vi "Cleanup.vi"(8 "error in (no error)":errorcluster, 11 "VISA GPS in":refnum<class "VISA GPS.lvclass">) -> (0 "error out":errorcluster)   [LabVIEW 2020, in "nmea.lvlib" / "VISA GPS.lvclass"]
uses:
  VISA GPS.lvclass
  VISA GPS.lvclass/VISA GPS.ctl
  nmea/nmea.lvclass
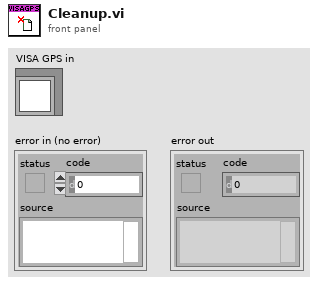
[diagram p1: front panel]
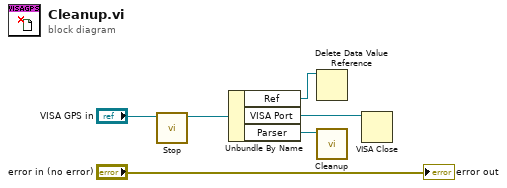
[diagram p0: block diagram]
diagram:
  n1 = call "Stop.vi"("VISA GPS in"="VISA GPS in") -> ("VISA GPS out"=w1:refnum<class "VISA GPS.lvclass">)  [unwired: 9 in, 1 out]
  n2 = Unbundle By Name(w1) -> ("Ref"=w5:refnum<data-value>, "VISA Port"=w4:refnum<visa-resource-name>, "Parser"=w3:refnum<class "nmea.lvclass">)
  n3 = Delete Data Value Reference(data value reference=w5) -> ()  [unwired: 1 in, 2 out]
  n4 = call "Cleanup.vi"("nmea in"=w3) -> ()  [unwired: 10 in, 1 out]
  n5 = VISA Close(VISA resource name=w4) -> ()  [unwired: 1 in, 1 out]
  "error out" <- "error in (no error)"
